vi "StripsBuilder.vi"(8 "Error IN":errorcluster caption="entrée d'erreur (pas d'erreur)", 10 "Global STRIPS":T1={"Strips number"=enum."1", "Y binning"=1, "Gap (%)"=0, "Init strips"=FALSE, "Strips updated"=TRUE, "max"=400.0} {"Gap (%)" max=100 step=1; "Y binning" min=1 step=1}, 11 "Global CAM":T2) -> (0 "Error OUT":errorcluster caption="sortie d'erreur")   [LabVIEW 2020]
uses:
  defTypeConfigs/stripConfigurationProto.ctl
  defTypeConfigs/globalCAM.ctl
  defTypeConfigs/globalSTRIPS.ctl
panel:
  out "Tableau":T3[](array[typedef])
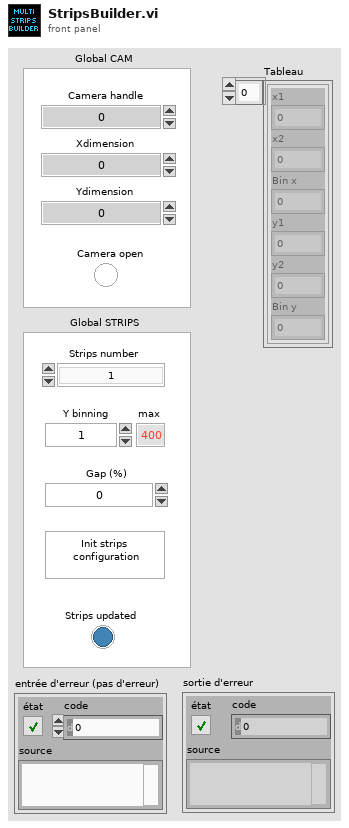
[diagram p1: front panel]
types:
  T1 = typedef "globalSTRIPS.ctl" = cluster{"Strips number":enum16{"12", "4", "2", "1"}, "Y binning":u32, "Gap (%)":u32, "Init strips":bool, "Strips updated":bool, "max":dbl}
  T2 = typedef "globalCAM.ctl" = cluster{"Ydimension":i32, "Xdimension":i32, "Camera handle":i32, "Camera open":bool}
  T3 = typedef "stripConfigurationProto.ctl" = cluster{"x1":u32, "x2":u32, "Bin x":u32, "y1":u32, "y2":u32, "Bin y":u32}
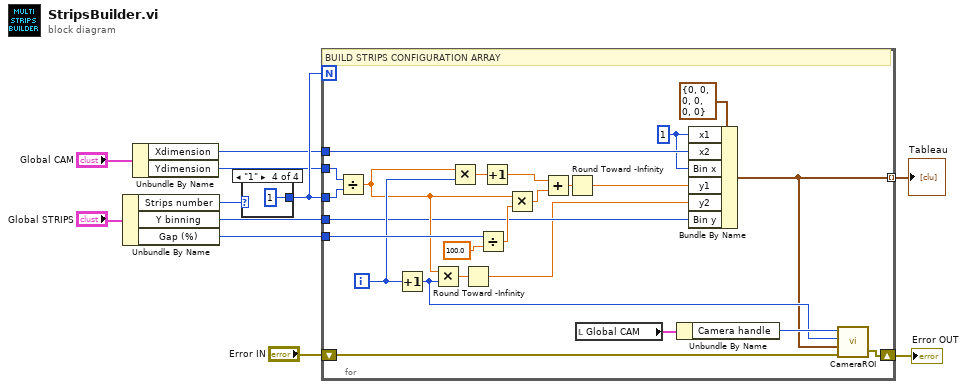
[diagram p0: block diagram]
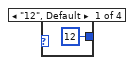
[diagram p2: hidden frame]
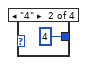
[diagram p3: hidden frame]
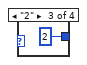
[diagram p4: hidden frame]
diagram:
  n1 = Unbundle By Name("Global STRIPS") -> ("Strips number"=w7:enum16{"12", "4", "2", "1"}, "Y binning"=w5:u32, "Gap (%)"=w6:u32)
  n2 = Unbundle By Name("Global CAM") -> ("Xdimension"=w3:i32, "Ydimension"=w4:i32)
  n3 = case shown="\"1\"" w7 {
    tunnel: [12 4 2 1] -> w8
    frame "12", Default {
    }
    frame "4" {
    }
    frame "2" {
    }
    frame "1" {
    }
  }
  n4 = for {
    N: w8 -> [_]
    tunnel: w3 -> [w38]
    tunnel: w4 -> [w36]
    tunnel: w5 -> [w24]
    tunnel: w8 -> [w35]
    tunnel: w6 -> [w33]
    tunnel: [w17] -> w9 mode=indexing
    shift-right: [w20] -> w10
    shift-left: "Error IN" -> [w21]
    i -> [w26]
    w37 = u32 1 ("x1")
    # "BUILD STRIPS CONFIGURATION ARRAY"
    n5 = Divide(x=w36, y=w35) -> (x/y=w25:dbl)
    n6 = Increment(x=w26) -> (x+1=w18:i32)
    n7 = Multiply(x=w25, y=w18) -> (x*y=w27:dbl)
    n8 = Multiply(x=w25, y=w26) -> (x*y=w30:dbl)
    n9 = Round Toward -Infinity(1:w27) -> (0:w22:dbl)
    n10 = Divide(x=w33, y=100.0) -> (x/y=w32:dbl)
    n11 = Increment(x=w30) -> (x+1=w29:dbl)
    n12 = Multiply(x=w25, y=w32) -> (x*y=w28:dbl)
    n13 = Add(x=w29, y=w28) -> (x+y=w31:dbl)
    n14 = Round Toward -Infinity(1:w31) -> (0:w23:dbl)
    n15 = local read "Global CAM"() -> (w16:T2)
    n16 = Unbundle By Name(w16) -> ("Camera handle"=w19:i32)
    n17 = Bundle By Name(cluster=T3 {"x1"=0, "x2"=0, "Bin x"=0, "y1"=0, "y2"=0, "Bin y"=0} ("Strip proto"), "x1"=w37, "x2"=w38, "Bin x"=w37, "y1"=w23, "y2"=w22, "Bin y"=w24) -> (w17:T3)
    n18 = call <userlib>:"CameraROI.vi"("error in"=w21, "ROI Params"=w17, "ROI Index"=w18, "Camera Handle"=w19) -> ("error out"=w20:errorcluster)  [unwired: 1 out]
  }
  "Error OUT" <- w10
  "Tableau" <- w9
